vi "iRobot Poll Sensor Group 1.vi"(8 "error in":errorcluster, 11 "UART port in":T4) -> (0 "error out":errorcluster, 1 "Timed Out?":bool, 2 "Sensor Group 1":T1, 3 "UART port out":T4)   [LabVIEW 2010]
doc: "Poll the iRobot for Sensor Group 1; blocks until response is received, or the operation has timed out.\n\nThis VI both writes to AND reads from the serial port.\n<b>NOTE</b>: This should not be used in a loop if other serial reading or writing VIs are called in parallel loops."
uses:
  UART/UART Port Type.ctl
  Sensor Controls/iRobot Sensor Group 1.ctl
  Sensor Controls/iRobot Bumps + Wheel Drops.ctl
  Sensor Controls/iRobot Low-Side Driver + Wheel Overcurrent.ctl
  Open Interface Controls/iRobot Sensor ID.ctl
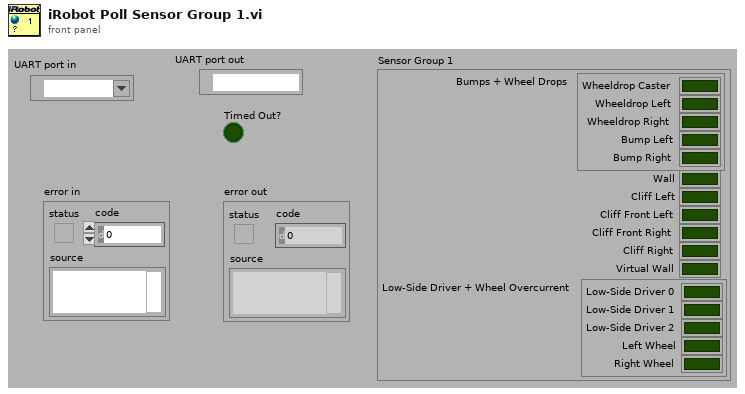
[diagram p1: front panel]
types:
  T1 = typedef "iRobot Sensor Group 1.ctl" = cluster{"Bumps + Wheel Drops":T2, "Wall":bool, "Cliff Left":bool, "Cliff Front Left":bool, "Cliff Front Right":bool, "Cliff Right":bool, "Virtual Wall":bool, "Low-Side Driver + Wheel Overcurrent":T3}
  T2 = typedef "iRobot Bumps + Wheel Drops.ctl" = cluster{"Wheeldrop Caster":bool, "Wheeldrop Left":bool, "Wheeldrop Right":bool, "Bump Left":bool, "Bump Right":bool}
  T3 = typedef "iRobot Low-Side Driver + Wheel Overcurrent.ctl" = cluster{"Low-Side Driver 0":bool, "Low-Side Driver 1":bool, "Low-Side Driver 2":bool, "Left Wheel":bool, "Right Wheel":bool}
  T4 = typedef "UART Port Type.ctl" = refnum<visa-resource-name>
  T5 = typedef "iRobot Sensor ID.ctl" = enum8{"Sensor Group 0", "Sensor Group 1", "Sensor Group 2", "Sensor Group 3", "Sensor Group 4", "Sensor Group 5", "Sensor Group 6", "Bump + Wheel Drop", "Wall", "Cliff Left", "Cliff Front Left", "Cliff Front Right", "Cliff Right", "Virtual Wall", "Low Side Driver + Wheel Overcurrent", "Unused 0", "Unused 1", "Infrared", "Buttons", "Distance", "Angle", "Charging State", "Voltage", "Current", "Battery Temperature", "Battery Charge", "Battery Capacity", "Wall Signal", "Cliff Left Signal", "Cliff Front Left Signal", "Cliff Front Right Signal", "Cliff Right Signal", "Cargo Bay Digital Inputs", "Cargo Bay Analog Signal", "Charging Sources Available", "OI Mode", "Song Number", "Song Playing", "Number of Stream Packets", "Requested Velocity", "Requested Radius", "Requested Right Velocity", "Requested Left Velocity"}
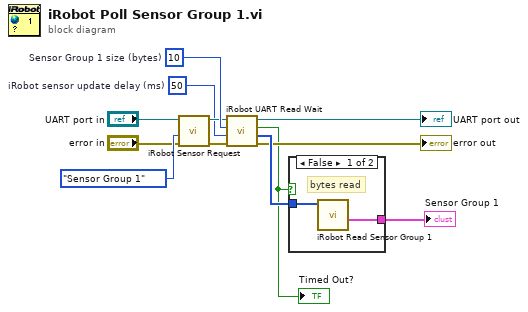
[diagram p0: block diagram]
diagram:
  w3 = 50  # iRobot sensor update delay (ms)
  w11 = 10  # Sensor Group 1 size (bytes)
  n1 = call "iRobot Sensor Request.vi"("error in"="error in", "Sensor ID"=iRobot_Sensor_ID."Sensor Group 1", "UART port in"="UART port in") -> ("error out"=w6:errorcluster, "UART port out"=w9:T4)  [unwired: 7 in]
  n2 = call "iRobot UART Read Wait.vi"("error in"=w6, "timeout (ms)"=w3, "Number of Bytes"=w11, "UART port in"=w9) -> ("error out"=→"error out":errorcluster, "UART Stream"=w10:u8[], "Timed Out?"=w2:bool, "UART port out"=→"UART port out":T4)  [unwired: 4 in]
  "Timed Out?" <- w2
  n3 = case shown="False" w2 {
    tunnel: w10 -> [w14 _]
    tunnel: [w13 _] -> w1
    frame False {
      # "bytes read"
      n4 = call "iRobot Read Sensor Group 1.vi"("stream in"=w14) -> ("Sensor Group 1"=w13:T1)  [unwired: 9 in, 1 out]
    }
    frame True {
      # "timeout"
    }
  }
  "Sensor Group 1" <- w1
